vi "Write Velocity (cnts_sec).vi"(8 "error in (no error)":errorcluster, 10 "Velocity (cnts/sec)":dbl=100.0, 11 "Filter Wheel Simulator in":refnum<class "Filter Wheel Simulator.lvclass">) -> (0 "error out":errorcluster, 3 "Filter Wheel Simulator out":refnum<class "Filter Wheel Simulator.lvclass">)   [LabVIEW 2021, in "Filter Wheel Simulator.lvclass"]
uses:
  Filter Wheel Simulator.lvclass
  Filter Wheel Simulator.lvclass/Filter Wheel Simulator.ctl
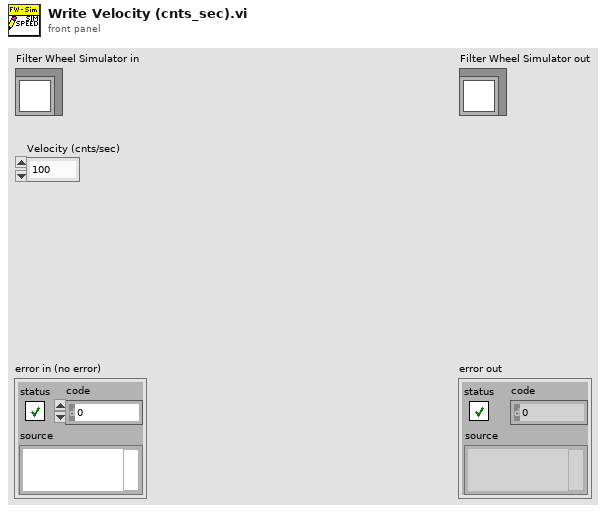
[diagram p1: front panel]
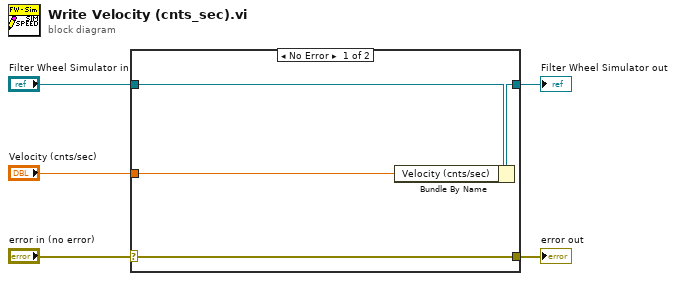
[diagram p0: block diagram]
diagram:
  n1 = case shown="No Error" "error in (no error)" {
    selector: "error in (no error)" -> [w9 w10]
    tunnel: [w9 w10] -> w4
    tunnel: [w7 w11] -> w2
    tunnel: "Filter Wheel Simulator in" -> [w8 w11]
    tunnel: "Velocity (cnts/sec)" -> [w6 _]
    frame No Error {
      n2 = Bundle By Name(cluster=w8, "Velocity (cnts/sec)"=w6) -> (w7:refnum<class "Filter Wheel Simulator.lvclass">)
    }
    frame Error {
    }
  }
  "error out" <- w4
  "Filter Wheel Simulator out" <- w2
